vi "create html.vi"(8 "error in (no error)":errorcluster caption="错误输入（无错误）", 10 "data":string[][](array[string]), 11 "columns":string[](array[string])) -> (0 "error out":errorcluster caption="错误输出", 3 "url":string)   [LabVIEW 2016, in "数据查询.lvlib"]
panel:
  out "结果字符串":string
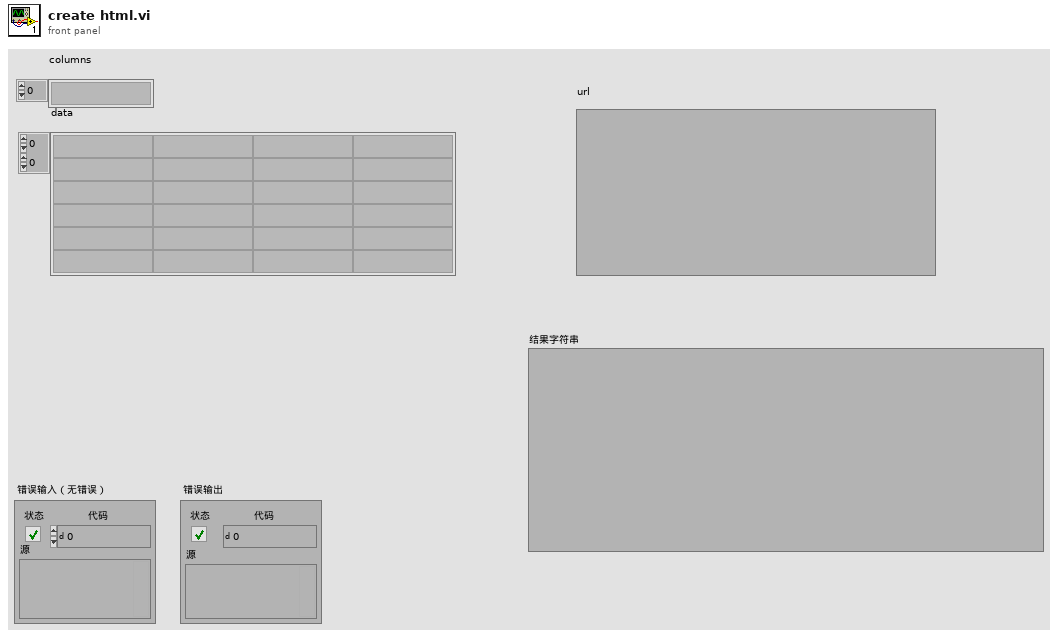
[diagram p1: front panel]
types:
  T1 = enum16{"open", "replace", "create", "open or create", "replace or create", "replace or create with confirmation"}
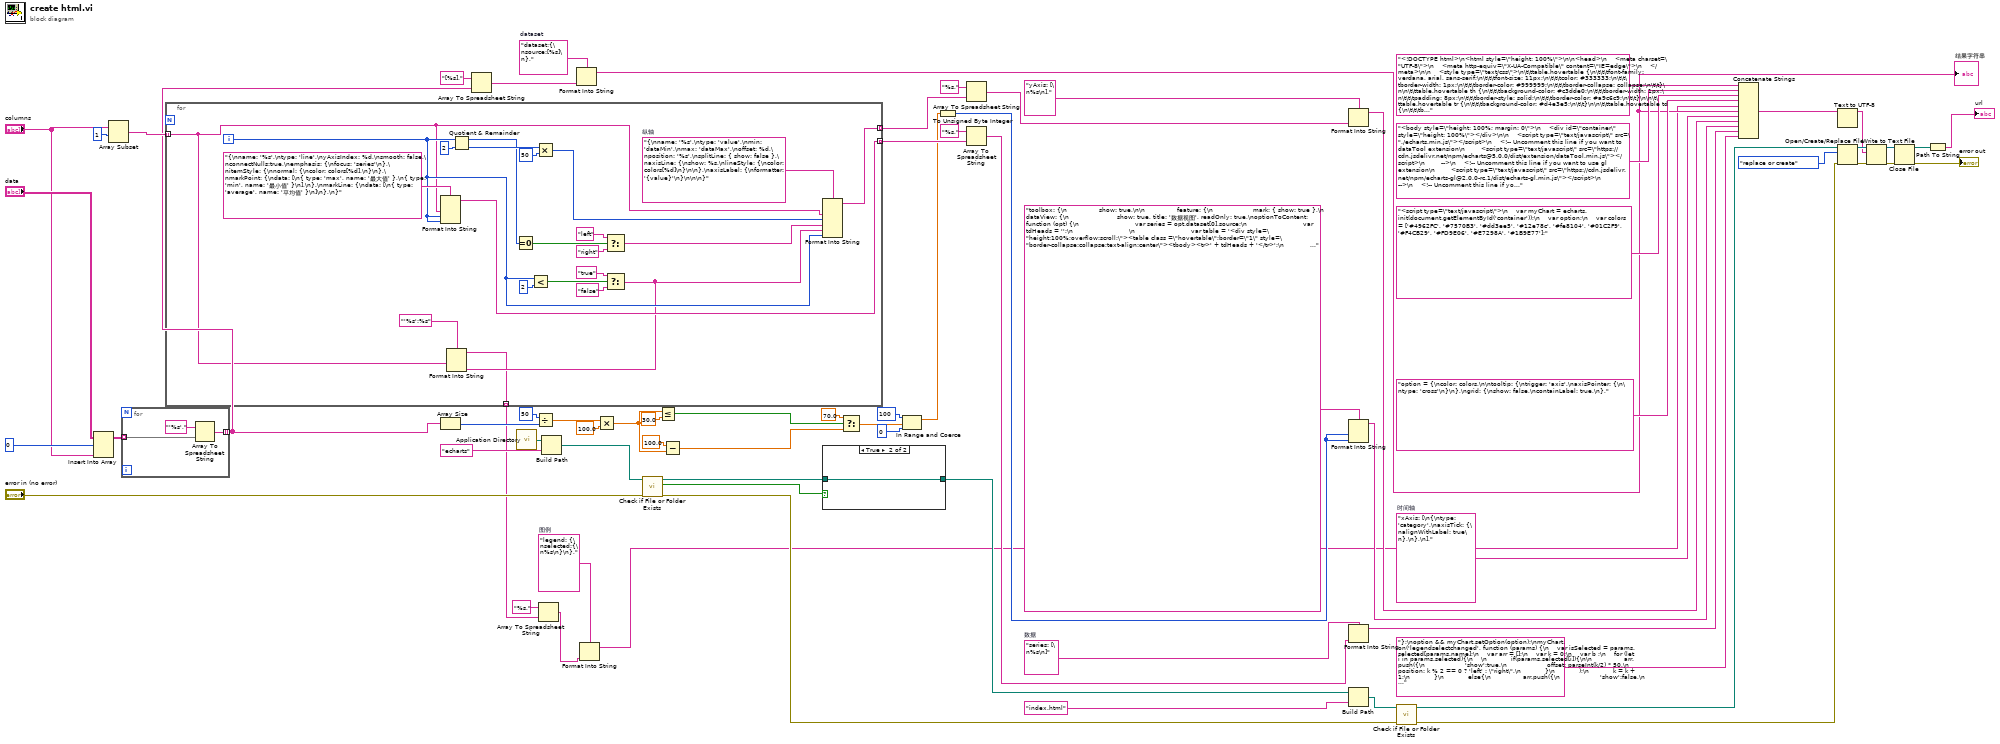
[diagram p0: block diagram]
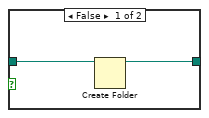
[diagram p2: hidden frame]
diagram:
  w2 = "legend: {\nselected:{\n%s\n}\n},"  # 图例
  w34 = "dataset:{\nsource:[%s]\n},"  # dataset
  w65 = "series: [\n%s\n]"  # 数据
  w32 = "xAxis: [\n{\ntype: 'category',\naxisTick: {\nalignWithLabel: true\n},\n},\n],"  # 时间轴
  n1 = Insert Into Array(array="data", index (row)=0 ("索引 (行)"), new element="columns") -> (w29:string[][])  [unwired: 1 in]
  n2 = Array Subset(array="columns", index=1 ("索引")) -> (w24:string[])  [unwired: 1 in]
  n3 = for {
    tunnel: w29 -> [w74] mode=indexing
    tunnel: [w72] -> w23 mode=indexing
    n4 = Array To Spreadsheet String(array=w74, 3:"'%s'," ("格式字符串")) -> (spreadsheet string=w72:string)  [unwired: 1 in]
  }
  n5 = for {
    tunnel: w24 -> [w77] mode=indexing
    tunnel: [w95] -> w61 mode=indexing
    tunnel: [w93] -> w58 mode=indexing
    tunnel: [w75] -> w4 mode=indexing
    i -> [w83]
    w96 = "{\nname: '%s',\ntype: 'value',\nmin: 'dataMin',\nmax: 'dataMax',\noffset: %d,\nposition: '%s',\nsplitLine: { show: false },\naxisLine: {\nshow: %s,\nlineStyle: {\ncolor: colors[%d]\n}\n\n},\naxisLabel: {\nformatter: '{value}'\n}\n\n\n}"  # 纵轴
    n6 = Format Into String(format string="{\nname: '%s',\ntype: 'line',\nyAxisIndex: %d,\nsmooth: false,\nconnectNulls:true,\nemphasis: {\nfocus: 'series'\n},\nitemStyle: {\nnormal: {\ncolor: colors[%d],\n}\n},\nmarkPoint: {\ndata: [\n{ type: 'max', name: '最大值' },\n{ type: 'min', name: '最小值' }\n],\n},\nmarkLine: {\ndata: [\n{ type: 'average', name: '平均值' }\n]\n},\n}", w77, w83, w83) -> (resulting string=w93:string)  [unwired: 2 in, 1 out]
    n7 = Quotient & Remainder(x=w83, y=2) -> (x-y*floor(x/y)=w88:i32, floor(x/y)=w91:i32)
    n8 = Equal To 0?(x=w88) -> (x = 0?=w87:bool)
    n9 = Less?(x=w83, y=2) -> (x < y?=w81:bool)
    n10 = Multiply(x=w91, y=50) -> (x*y=w89:i32)
    n11 = Select(t="left", s=w87, f="right") -> (s? t:f=w84:string)
    n12 = Select(t="true", s=w81, f="false") -> (s? t:f=w76:string)
    n13 = Format Into String(format string="'%s':%s" ("格式字符串"), w77, w76) -> (resulting string=w75:string)  [unwired: 2 in, 1 out]
    n14 = Format Into String(format string=w96, w77, w89, w84, w76, w83) -> (resulting string=w95:string)  [unwired: 2 in, 1 out]
  }
  n15 = Array Size(array=w23) -> (size(s)=w22:i32)
  n16 = Array To Spreadsheet String(array=w23, 3:"[%s]," ("格式字符串")) -> (spreadsheet string=w31:string)  [unwired: 1 in]
  n17 = call <vilib>:"Application Directory.vi"() -> ("Application Directory"=w56:path)
  n18 = Divide(x=50, y=w22) -> (x/y=w20:dbl)
  n19 = Array To Spreadsheet String(array=w4, 3:"%s," ("格式字符串")) -> (spreadsheet string=w3:string)  [unwired: 1 in]
  n20 = Build Path(base path=w56, name or relative path="echarts" ("名称或相对路径")) -> (appended path=w54:path)
  n21 = Format Into String(format string=w34, w31) -> (resulting string=w30:string)  [unwired: 2 in, 1 out]
  "结果字符串" <- w30
  n22 = Format Into String(format string=w2, w3) -> (resulting string=w1:string)  [unwired: 2 in, 1 out]
  n23 = Multiply(x=w20, y=100.0) -> (x*y=w11:dbl)
  n24 = call <vilib>:"Check if File or Folder Exists.vi"("error in (no error)"="error in (no error)", "path"=w54) -> ("error out"=w46:errorcluster, "file or folder exists?"=w53:bool, "dup path"=w52:path)  [unwired: 7 in]
  n25 = Less Or Equal?(x=w11, y=30.0) -> (x <= y?=w9:bool)
  n26 = Subtract(x=100.0, y=w11) -> (x-y=w7:dbl)
  n27 = case shown="True" w53 {
    tunnel: w52 -> [w98 w99]
    tunnel: [w97 w99] -> w51
    frame False {
      n28 = Create Folder(path (use dialog)=w98) -> (created path=w97:path)  [unwired: 2 in, 2 out]
    }
    frame True {
    }
  }
  n29 = Select(t=70.0, s=w9, f=w7) -> (s? t:f=w6:dbl)
  n30 = In Range and Coerce(upper limit=100, x=w6, lower limit=0) -> (coerced(x)=w15:dbl)  [unwired: 1 out]
  n31 = To Unsigned Byte Integer(number=w15) -> (unsigned 8bit integer=w12:u8)
  n32 = Array To Spreadsheet String(array=w61, 3:"%s," ("格式字符串")) -> (spreadsheet string=w60:string)  [unwired: 1 in]
  n33 = Array To Spreadsheet String(array=w58, 3:"%s," ("格式字符串")) -> (spreadsheet string=w57:string)  [unwired: 1 in]
  n34 = Format Into String(format string="yAxis: [\n%s\n],", w60) -> (resulting string=w66:string)  [unwired: 2 in, 1 out]
  n35 = Format Into String(format string="toolbox: {\n                show: true,\n\n                feature: {\n                    mark: { show: true },\n                    dataView: {\n                        show: true, title: '数据视图', readOnly: true,\noptionToContent: function (opt) {\n                            var series = opt.dataset[0].source;\n                            var tdHeads = '';\n                            \n                            var table = '<div style=\"height:100%;overflow:scroll;\"><table class =\"hovertable\";border=\"1\" style=\"border-collapse:collapse;text-align:center\"><tbody><tr>' + tdHeads + '</tr>';\n                            var tdBodys = '';\n                            for (var i = 0, l = series.length; i < l; i++) {\n                                for (var j = 0; j < series[0].length; j++) {\n                                    if (typeof (series[i][j]) == 'object') {\n\n \n                                        tdBodys += '<td>' + series[i][j] + '</td>';\n                                    } else {\n                                        tdBodys += '<td>' + series[i][j] + '</td>';\n                                    }\n                                }\n                                table += '<tr onmouseover=\"this.style.backgroundColor=&#39;#ffff66&#39;;\" onmouseout=\"this.style.backgroundColor=&#39;#d4e3e5&#39;;\" style=\"background-color: rgb(212, 227, 229);\">' + tdBodys + '</tr>';\n                                tdBodys = '';\n                            }\n                            table += '</tbody></table></div>';\n                            return table;\n                        }\n                    },\n                    magicType: { show: true, title: { line: '折线图', bar: '柱状图', }, type: ['line', 'bar'] },\n                    restore: { show: true, title: '刷新' },\n                    saveAsImage: { show: true, title: '保存图片', backgroundColor: '#fff' },\n                }\n            },\n\n\ndataZoom: [ { show: true, type: 'slider' , realtime: true, start: %d, end: 100, height: 50,\n                bottom: 10, }, { type: 'inside' , start: %d, end: 100 }, ],", w12, w12) -> (resulting string=w13:string)  [unwired: 2 in, 1 out]
  n36 = Format Into String(format string=w65, w57) -> (resulting string=w64:string)  [unwired: 2 in, 1 out]
  n37 = Build Path(base path=w51, name or relative path="index.html" ("名称或相对路径")) -> (appended path=w49:path)
  n38 = call <vilib>:"Check if File or Folder Exists.vi"("error in (no error)"=w46, "path"=w49) -> ("error out"=w47:errorcluster, "dup path"=w48:path)  [unwired: 7 in, 1 out]
  n39 = Concatenate Strings("<!DOCTYPE html>\n<html style=\"height: 100%\">\n\n<head>\n    <meta charset=\"UTF-8\">\n    <meta http-equiv=\"X-UA-Compatible\" content=\"IE=edge\">\n    </meta>\n\n    <style type=\"text/css\">\n\t\ttable.hovertable {\n\t\t\tfont-family: verdana, arial, sans-serif;\n\t\t\tfont-size: 11px;\n\t\t\tcolor: #333333;\n\t\t\tborder-width: 1px;\n\t\t\tborder-color: #999999;\n\t\t\tborder-collapse: collapse;\n\t\t}\n\n\t\ttable.hovertable th {\n\t\t\tbackground-color: #c3dde0;\n\t\t\tborder-width: 1px;\n\t\t\tpadding: 8px;\n\t\t\tborder-style: solid;\n\t\t\tborder-color: #a9c6c9;\n\t\t}\n\n\t\ttable.hovertable tr {\n\t\t\tbackground-color: #d4e3e5;\n\t\t}\n\n\t\ttable.hovertable td {\n\t\t\tborder-width: 1px;\n\t\t\tpadding: 8px;\n\t\t\tborder-style: solid;\n\t\t\tborder-color: #a9c6c9;\n\t\t}\n\t</style>\n</head>", "<body style=\"height: 100%; margin: 0\">\n    <div id=\"container\" style=\"height: 100%\"></div>\n\n    <script type=\"text/javascript\" src=\"./echarts.min.js\"></script>\n    <!-- Uncomment this line if you want to dataTool extension\n        <script type=\"text/javascript\" src=\"https://cdn.jsdelivr.net/npm/echarts@5.0.0/dist/extension/dataTool.min.js\"></script>\n        -->\n    <!-- Uncomment this line if you want to use gl extension\n        <script type=\"text/javascript\" src=\"https://cdn.jsdelivr.net/npm/echarts-gl@2.0.0-rc.1/dist/echarts-gl.min.js\"></script>\n        -->\n    <!-- Uncomment this line if you want to echarts-stat extension\n        <script type=\"text/javascript\" src=\"https://cdn.jsdelivr.net/npm/echarts-stat@latest/dist/ecStat.min.js\"></script>\n        -->\n    <!-- Uncomment this line if you want to use map\n        <script type=\"text/javascript\" src=\"https://cdn.jsdelivr.net/npm/echarts@5.0.0/map/js/china.js\"></script>\n        <script type=\"text/javascript\" src=\"https://cdn.jsdelivr.net/npm/echarts@5.0.0/map/js/world.js\"></script>\n        -->\n    <!-- Uncomment these two lines if you want to use bmap extension\n        <script type=\"text/javascript\" src=\"https://api.map.baidu.com/api?v=2.0&ak=<Your Key Here>\"></script>\n        <script type=\"text/javascript\" src=\"https://cdn.jsdelivr.net/npm/echarts@5.0.0/dist/extension/bmap.min.js\"></script>\n        -->", "<script type=\"text/javascript\">\n    var myChart = echarts.init(document.getElementById('container'));\n    var option;\n    var colors = ['#4962FC', '#7570B3', '#dd3ee5', '#12e78c', '#fe8104', '#01C2F9', '#F4CB29', '#FD9E06', '#E7298A', '#1B9E77'];", "option = {\ncolor: colors,\n\ntooltip: {\ntrigger: 'axis',\naxisPointer: {\n\ntype: 'cross'\n}\n},\ngrid: {\nshow: false,\ncontainLabel: true,\n},", w1, w30, w32, w66, w13, w64, "};\noption && myChart.setOption(option);\nmyChart.on('legendselectchanged', function (params) {\n    var isSelected = params.selected[params.name];\n    var arr = [];\n    var k = 0;\n    var b ;\n    for (let i in params.selected){\n    \n            if(params.selected[i]){\n\n                arr.push({\n                    'show':true,\n                    offset: parseInt(k/2) * 50,\n                    position: k % 2 == 0 ? 'left' : \"right\",\n            }\n            );\n            k = k + 1;\n            }\n            else{\n                arr.push({\n                    'show':false,\n                    offset: 0,\n                });\n            }\n    };\nb = {yAxis:JSON.parse(JSON.stringify(arr))};\n    option && myChart.setOption(b);\n});\n</script>\n</body>\n\n</html>") -> (w36:string)
  n40 = Text to UTF-8(11:w36) -> (3:w35:string)  [unwired: 2 in, 1 out]
  n41 = Open/Create/Replace File(file path (use dialog)=w48, error in=w47, operation (0:open)=T1."replace or create" ("操作(0:open)")) -> (refnum out=w42:refnum<file>, error out=w43:errorcluster)  [unwired: 3 in, 1 out]
  n42 = Write to Text File(file (use dialog)=w42, text=w35, error in=w43) -> (refnum out=w41:refnum<file>, error out=w40:errorcluster)  [unwired: 1 in, 1 out]
  n43 = Close File(refnum=w41, error in=w40) -> (path=w39:path, error out=→"error out":errorcluster)
  n44 = Path To String(path=w39) -> (string=→"url":string)
